vi "Get Targets_Do.vi"(8 "error in (no error)":errorcluster, 11 "Dependency Source_Custom in":refnum<class "Dependency Source_Custom.lvclass">) -> (0 "error out":errorcluster, 1 "Success?":bool, 2 "External Target Map":map{string, string}(c390), 3 "Internal Target Map":map{string, string}(c390), 4 "Unhandled Targets":string[](array[string]))   [LabVIEW 2019, in "Project.Dependencies Finder.lvlib" / "Dependency Source_Custom.lvclass"]
doc: "Get internal and external targets for the dependency source.\n\nReturns the data from the class."
uses:
  Dependency Source_Custom.lvclass
  C:/Current projects/LV32.2019..ProjectDependenciesFinder/Dependency Source/Dependency Source.lvclass
  Dependency Source_Custom.lvclass/Dependency Source_Custom.ctl
  Dependency Source/Dependency Source.lvclass
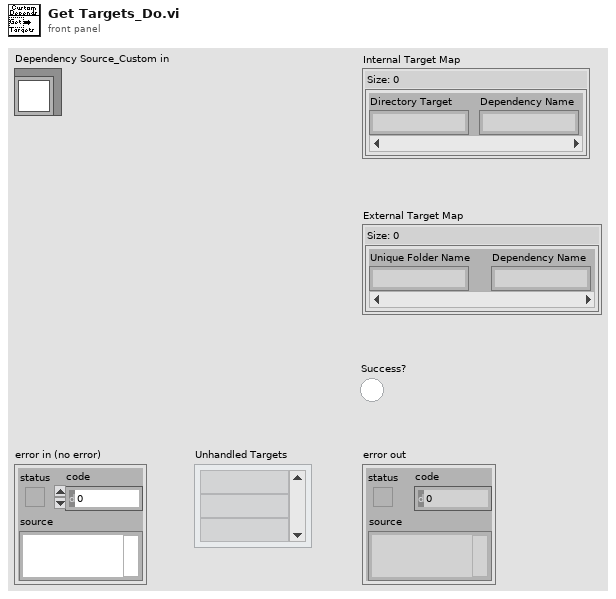
[diagram p1: front panel]
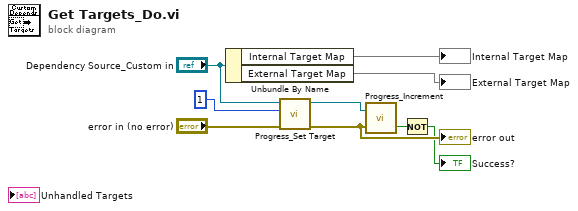
[diagram p0: block diagram]
diagram:
  n1 = Unbundle By Name("Dependency Source_Custom in") -> ("Internal Target Map"=→"Internal Target Map":map{string, string}, "External Target Map"=→"External Target Map":map{string, string})
  n2 = call "Progress_Set Target.vi"("error in (no error)"="error in (no error)", "Set Target"=1, "Dependency Source in"="Dependency Source_Custom in") -> ("error out"=w3:errorcluster, "Dependency Source out"=w7:refnum<class "Dependency Source_Custom.lvclass">)  [unwired: 7 in]
  "error out" <- w3
  n3 = call "Progress_Increment.vi"("error in (sync)"=w3, "Dependency Source in"=w7) -> ("Abort?"=w2:bool)  [unwired: 1 out]
  n4 = Not(x=w2) -> (.not. x?=→"Success?":bool)
